vi "Event-Start.vi"(8 "error in (no error)":errorcluster, 10 "Data ref. in":refnum<data-value>, 11 "UI ref. in":refnum<data-value>) -> (0 "error out":errorcluster, 2 "Data ref.":refnum<data-value>, 3 "UI ref.":refnum<data-value>)   [LabVIEW 2013, in "CameraVision.lvlib" / "CV-UI.lvclass"]
uses:
  CV-UI.lvclass
  Main/CV-Main.lvclass
  CV-UI.lvclass/CV-UI.ctl
  Main/Main-actions.ctl
  Read Acquisition.vi
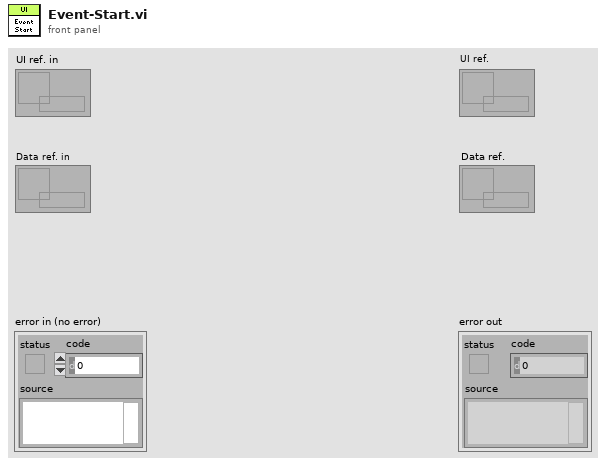
[diagram p1: front panel]
types:
  T1 = typedef "CameraVision.lvlib/CV-Main.lvclass/Main-actions.ctl" = enum16{"Idle", "Initialize", "Load defaults", "Update settings", "Check settings", "Save settings", "Save settings with dialog", "Load settings", "Load data", "Activate", "Start", "Wait for start signal", "Acquire & process", "Iterate", "Stop", "Refresh display", "Refresh status", "View camera settings", "View grabber settings", "Exit"}
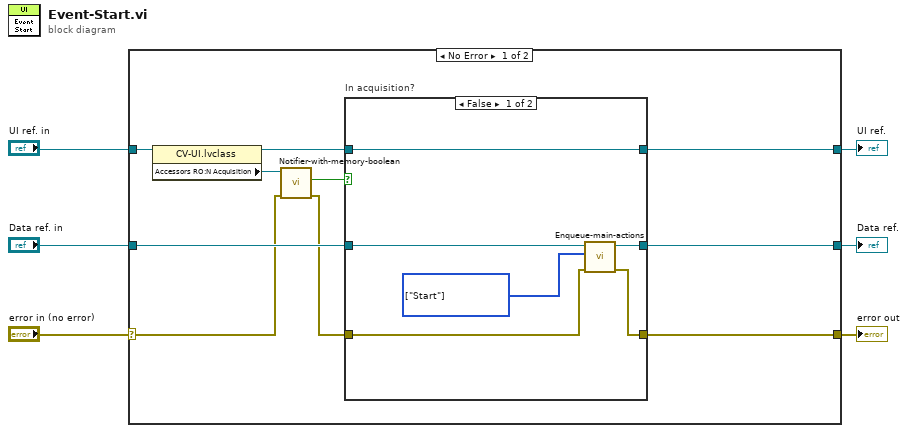
[diagram p0: block diagram]
diagram:
  n1 = case shown="No Error" "error in (no error)" {
    selector: "error in (no error)" -> [w8 w28]
    tunnel: [w13 w28] -> w5
    tunnel: [w16 w27] -> w3
    tunnel: "UI ref. in" -> [w14 w27]
    tunnel: "Data ref. in" -> [w11 w26]
    tunnel: [w15 w26] -> w1
    frame No Error {
      n2 = property class="CV-UI.lvclass"(reference=w14) -> (reference out=w12:refnum<data-value>, "Accessors RO:N Acquisition"=w10:refnum<notifier>)  [unwired: 1 in, 1 out]
      n3 = call "Notifier-with-memory-boolean.vi"("error in"=w8, "Notifier in"=w10) -> ("error IO"=w9:errorcluster, "Notification"=w7:bool)  [unwired: 8 in]
      n4 = case "In acquisition?" shown="False" w7 {
        tunnel: w12 -> [w22 w24]
        tunnel: w11 -> [w17 w25]
        tunnel: [w22 w24] -> w16
        tunnel: [w18 w25] -> w15
        tunnel: w9 -> [w20 w23]
        tunnel: [w19 w23] -> w13
        frame False {
          w21 = T1[] [enum."Start"] items=["Idle", "Initialize", "Load defaults", "Update settings", "Check settings", "Save settings", "Save settings with dialog", "Load settings", "Load data", "Activate", "Start", "Wait for start signal", "Acquire & process", "Iterate", "Stop", "Refresh display", "Refresh status", "View camera settings", "View grabber settings", "Exit"] ("State array")
          n5 = call "Enqueue-main-actions.vi"("error in (no error)"=w20, "State array"=w21, "Data ref. in"=w17) -> ("error out"=w19:errorcluster, "Data ref."=w18:refnum<data-value>)  [unwired: 6 in, 1 out]
        }
        frame True {
        }
      }
    }
    frame Error {
    }
  }
  "error out" <- w5
  "Data ref." <- w1
  "UI ref." <- w3
